vi "Get Properties by Item GUID.vi"(8 "Error In":errorcluster, 11 "Item References":T1[](array[typedef]) format="%.0x") -> (0 "Error Out":errorcluster, 2 "Properties and Values []":string[][](array[string]))   [LabVIEW 2017]
uses:
  <vilib>/NI Veristand/Custom Device API/Custom Device Item Ref.ctl
  NationalInstruments.VeriStand.SystemStorage
  <vilib>/NI Veristand/Custom Device API/Custom Device API.lvlib
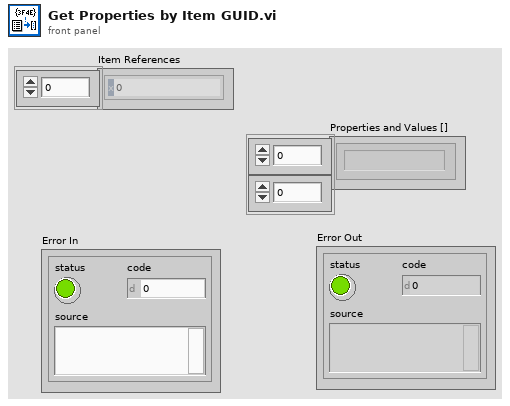
[diagram p1: front panel]
types:
  T1 = typedef "Custom Device API.lvlib/Custom Device Item Ref.ctl" = u64
  T2 = typedef "Custom Device API.lvlib/Custom Device Pointer.ctl" = refnum<k24>
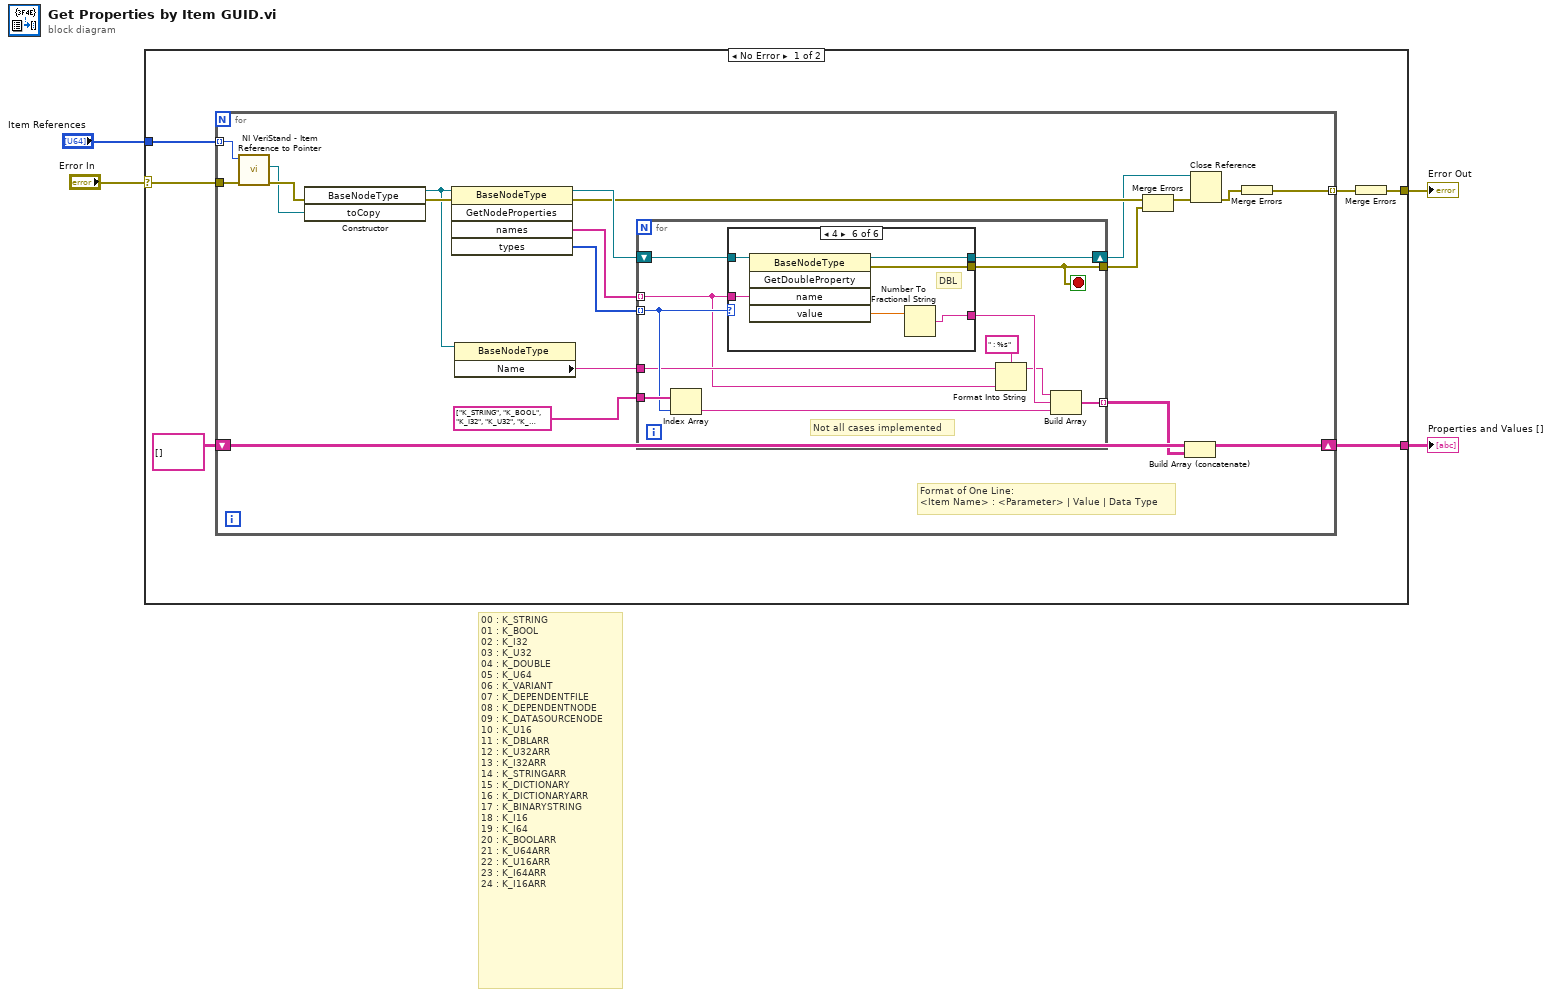
[diagram p0: block diagram]
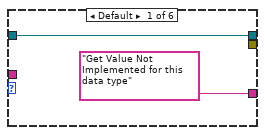
[diagram p2: hidden frame]
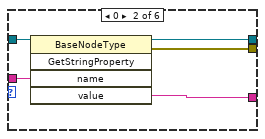
[diagram p3: hidden frame]
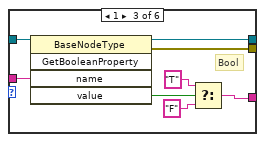
[diagram p4: hidden frame]
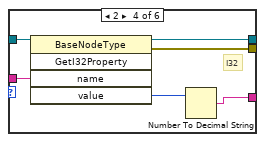
[diagram p5: hidden frame]
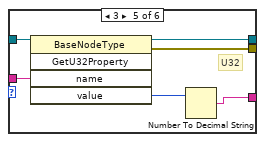
[diagram p6: hidden frame]
diagram:
  # "00 : K_STRING\n01 : K_BOOL\n02 : K_I32\n03 : K_U32\n04 : K_DOUBLE\n05 : K_U64\n06 : K_VARIANT\n07 : K_DEPENDENTFILE\n08 : K_DEPENDENTNODE\n09 : K_DATASOURCENODE\n10 : K_U16\n11 : K_DBLARR\n12 : K_U32ARR\n13 : K_I32ARR\n14 : K_STRINGARR\n15 : K_DICTIONARY\n16 : K_DICTIONARYARR\n17 : K_BINARYSTRING\n18 : K_I16\n19 : K_I64\n20 : K_BOOLARR\n21 : K_U64ARR\n22 : K_U16ARR\n23 : K_I64ARR\n24 : K_I16ARR"
  n1 = case shown="No Error" "Error In" {
    selector: "Error In" -> [w9 w76]
    tunnel: [w8 w76] -> w3
    tunnel: [w6 _] -> w2
    tunnel: "Item References" -> [w5 _]
    frame No Error {
      n2 = for {
        tunnel: w9 -> [w30]
        tunnel: [w12] -> w10 mode=indexing
        shift-right: [w27] -> w6
        shift-left: string[][] [] -> [w28]
        tunnel: w5 -> [w26] mode=indexing
        # "Format of One Line:\n<Item Name> : <Parameter> | Value | Data Type"
        n3 = call <vilib>:"NI VeriStand - Item Reference to Pointer.vi"("error in (no error)"=w30, "Item Ref in"=w26) -> ("error out"=w13:errorcluster, "Node Pointer"=w11:T2)  [unwired: 6 in, 2 out]
        n4 = constructor class="BaseNodeType"(error in=w13, "toCopy"=w11) -> (reference out=w18:refnum<k24>, error out=w25:errorcluster)  [unwired: 2 in, 2 out]
        n5 = invoke class="BaseNodeType" method="GetNodeProperties"(reference=w18, error in=w25) -> (reference out=w23:refnum<k24>, error out=w22:errorcluster, "names"=w21:string[], "types"=w20:i32[])  [unwired: 3 in, 1 out]
        n6 = property class="BaseNodeType"(reference=w18) -> ("Name"=w17:string)  [unwired: 1 in, 2 out]
        n7 = for {
          tunnel: w21 -> [w34] mode=indexing
          tunnel: w20 -> [w40] mode=indexing
          tunnel: string[] ["K_STRING", "K_BOOL", "K_I32", "K_U32", "K_DOUBLE", "K_U64", "K_VARIANT", "K_DEPENDENTFILE", "K_DEPENDENTNODE", "K_DATASOURCENODE", "K_U16", "K_DBLARR", "K_U32ARR", "K_I32ARR", "K_STRINGARR", "K_DICTIONARY", "K_DICTIONARYARR", "K_BINARYSTRING", "K_I16", "K_I64", "K_BOOLARR", "K_U64ARR", "K_U16ARR", "K_I64ARR", "K_I16ARR"] ("Strings []") -> [w42]
          shift-right: [w37] -> w14
          shift-left: w23 -> [w41]
          tunnel: [w38] -> w16 mode=indexing
          tunnel: [w36] -> w19
          tunnel: w17 -> [w35]
          stop <- w36 stop-if-true
          # "Not all cases implemented"
          n8 = Index Array(array=w42, index=w40) -> (element=w31:string)
          n9 = case shown="4" w40 {
            tunnel: w41 -> [w44 w49 w57 w63 w69 w75]
            tunnel: w34 -> [_ w48 w56 w62 w68 w74]
            tunnel: ["Get Value Not Implemented for this data type" ("value") w47 w52 w58 w64 w70] -> w39
            tunnel: [w44 w46 w55 w61 w67 w73] -> w37
            tunnel: [_ w45 w54 w60 w66 w72] -> w36
            frame Default {
            }
            frame 0 {
              n10 = invoke class="BaseNodeType" method="GetStringProperty"(reference=w49, "name"=w48) -> (reference out=w46:refnum<k24>, error out=w45:errorcluster, "value"=w47:string)  [unwired: 3 in, 2 out]
            }
            frame 1 {
              # "Bool"
              n11 = invoke class="BaseNodeType" method="GetBooleanProperty"(reference=w57, "name"=w56) -> (reference out=w55:refnum<k24>, error out=w54:errorcluster, "value"=w53:bool)  [unwired: 3 in, 2 out]
              n12 = Select(t="T" ("GUID"), s=w53, f="F" ("GUID")) -> (s? t:f=w52:string)
            }
            frame 2 {
              # "I32"
              n13 = invoke class="BaseNodeType" method="GetI32Property"(reference=w63, "name"=w62) -> (reference out=w61:refnum<k24>, error out=w60:errorcluster, "value"=w59:i32)  [unwired: 3 in, 2 out]
              n14 = Number To Decimal String(number=w59) -> (decimal integer string=w58:string)  [unwired: 1 in]
            }
            frame 3 {
              # "U32"
              n15 = invoke class="BaseNodeType" method="GetU32Property"(reference=w69, "name"=w68) -> (reference out=w67:refnum<k24>, error out=w66:errorcluster, "value"=w65:u32)  [unwired: 3 in, 2 out]
              n16 = Number To Decimal String(number=w65) -> (decimal integer string=w64:string)  [unwired: 1 in]
            }
            frame 4 {
              # "DBL"
              n17 = invoke class="BaseNodeType" method="GetDoubleProperty"(reference=w75, "name"=w74) -> (reference out=w73:refnum<k24>, error out=w72:errorcluster, "value"=w71:dbl)  [unwired: 3 in, 2 out]
              n18 = Number To Fractional String(number=w71) -> (F-format string=w70:string)  [unwired: 3 in]
            }
          }
          n19 = Format Into String(format string=" : %s", initial string=w35, w34) -> (resulting string=w33:string)  [unwired: 1 in, 1 out]
          n20 = Build Array(w33, w39, w31) -> (w38:string[])
        }
        n21 = Merge Errors(w22, w19) -> (w24:errorcluster)
        n22 = Build Array (concatenate)(w28, w16) -> (w27:string[][])
        n23 = Close Reference(reference=w14, error in (no error)=w24) -> (error out=w29:errorcluster)
        n24 = Merge Errors(w29) -> (w12:errorcluster)
      }
      n25 = Merge Errors(w10) -> (w8:errorcluster)
    }
    frame Error {
    }
  }
  "Error Out" <- w3
  "Properties and Values []" <- w2
